vi "Move To Position According to List.vi"() -> ()   [LabVIEW 2020]
uses:
  Labview Library/Libraries/Basic Experiment/AutoTrace Element Result.ctl
  <vilib>/Analysis/coordinate.llb/3D Coordinate Conversion (Scalar).vi
  <vilib>/Utility/file.llb/Read Delimited Spreadsheet (string).vi
  Labview Library/Libraries/Read TDMS Data/Library/Read TDMS Data.lvlib
  Labview Library/Libraries/Basic Experiment/Basic Experiment.lvlib
  Labview Library/Libraries/Shift_Correction/Libraries/Shift_Correction/Shift_Correction.lvlib
  <vilib>/Analysis/NI_AALPro.lvlib
panel:
  out "Amp Difference":dbl=0.263119271037894
  out "Angle Difference (deg)":dbl=-0.09953145598427682
  out "AutoTrace Result":T1={"Pure Count"=497997.60921836324, "BackGround"=54839.90103535615, "AutoTrace File Path"=path "G:/Raw Data/AutoFocus/XY Graph/2024-03/AF XY 2024-03-21_205701.png", "Light Spot Pos"=[5.049998165058289, 143.35743224656605, 69.90496826]}
  in  "ColorCenter List Path":path=path "G:/Exp_Log/2024_02_12_ChargeDetection2/Accurate_LightSpot.csv"
  out "Table":string[][](array[string])
  in  "Index":u32=3
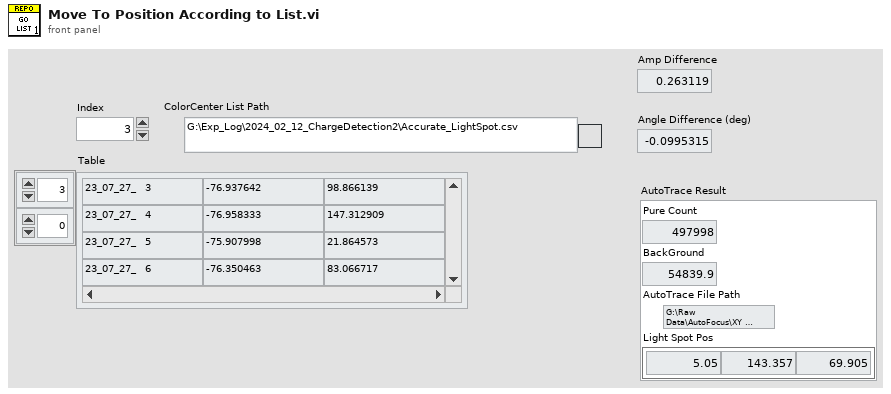
[diagram p1: front panel]
types:
  T1 = typedef "Basic Experiment.lvlib/AutoTrace Element Result.ctl" = cluster{"Pure Count":dbl, "BackGround":dbl, "AutoTrace File Path":path, "Light Spot Pos":dbl[]}
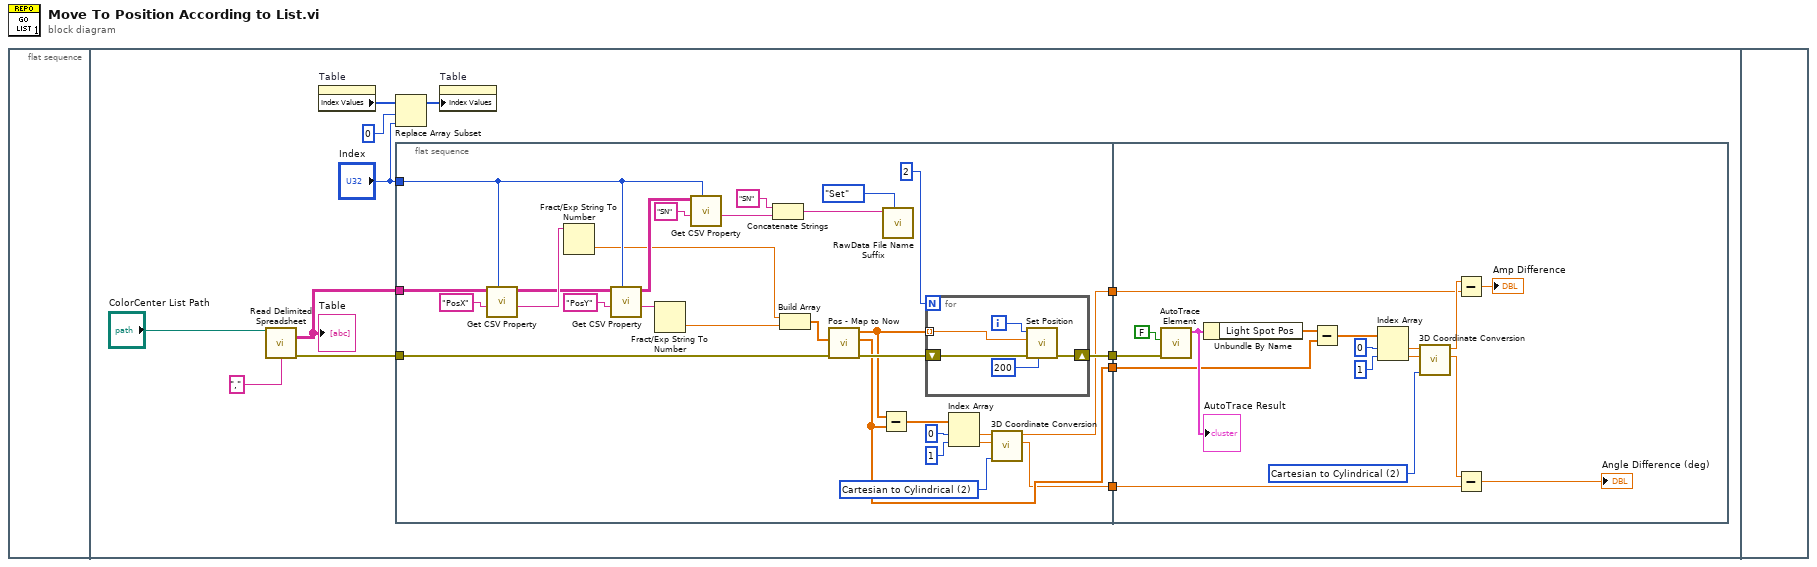
[diagram p0: block diagram]
diagram:
  n1 = flat-sequence {
    frame #0 {
    }
    frame #1 {
      n2 = call-poly <vilib>:"Read Delimited Spreadsheet.vi"("file path (dialog if empty)"="ColorCenter List Path", "delimiter (\\t)"="," ("delimiter (\\t)")) -> ("all rows"=w9:string[][], "error out"=w11:errorcluster)  [unwired: 8 in, 4 out]
      "Table" <- w9
      n3 = property on="Table" class="Arr (strict)"() -> ("Index Values"=w8:u32[])  [unwired: 2 in, 2 out]
      n4 = Replace Array Subset(array=w8, new element="Index", index=0) -> (w6:u32[])
      n5 = flat-sequence {
        tunnel: [w23] -> w4
        tunnel: w11 -> [w25]
        tunnel: "Index" -> [w34]
        tunnel: w9 -> [w41]
        tunnel: [w15] -> w3
        tunnel: [w14] -> w2
        tunnel: [w13] -> w1
        tunnel: w4 -> [w64]
        tunnel: w3 -> [w60]
        tunnel: w2 -> [w52]
        tunnel: w1 -> [w50]
        frame #0 {
          w16 = u16 2 items=["Cartesian to Spherical", "Spherical to Cartesian", "Cartesian to Cylindrical", "Cylindrical to Cartesian", "Spherical to Cylindrical", "Cylindrical to Spherical"] ("conversion type")
          n6 = call "Get CSV Property.vi"("Index"=w34, "Property Name"="PosX", "csv"=w41) -> ("Property value"=w40:string, "csv output"=w39:string[][])  [unwired: 7 in]
          n7 = Fract/Exp String To Number(string=w40) -> (number=w29:dbl)  [unwired: 3 in, 1 out]
          n8 = call "Get CSV Property.vi"("Index"=w34, "Property Name"="PosY", "csv"=w39) -> ("Property value"=w38:string, "csv output"=w36:string[][])  [unwired: 7 in]
          n9 = Fract/Exp String To Number(string=w38) -> (number=w28:dbl)  [unwired: 3 in, 1 out]
          n10 = call "Get CSV Property.vi"("Index"=w34, "Property Name"="SN", "csv"=w36) -> ("Property value"=w31:string)  [unwired: 7 in, 1 out]
          n11 = Concatenate Strings("SN" ("string"), w31) -> (w30:string)
          n12 = Build Array(w29, w28) -> (w26:dbl[])
          n13 = call "Pos - Map to Now.vi"("error in"=w25, "Goal Map Position"=w26) -> ("error out"=w24:errorcluster, "Marker Position Now"=w15:dbl[], "Goal Now Position"=w20:dbl[])  [unwired: 6 in, 1 out]
          n14 = Subtract(x=w20, y=w15) -> (x-y=w19:dbl[])
          n15 = call "RawData File Name Suffix.vi"("Mode"=enum16{"Set", "Get"}."Set", "Suffix"=w30) -> ()  [unwired: 9 in, 1 out]
          n16 = for {
            N: 2 -> [_]
            tunnel: w20 -> [w47] mode=indexing
            shift-right: [w45] -> w23
            shift-left: w24 -> [w44]
            i -> [w46]
            n17 = call "Set Position.vi"("Idle After Moving (ms)"=200, "error in"=w44, "Position"=w47, "Axis"=w46) -> ("error out"=w45:errorcluster)  [unwired: 7 in]
          }
          n18 = Index Array(array=w19, index #1=0 ("index"), index #2=1 ("index")) -> (element #1=w18:dbl, element #2=w17:dbl)
          n19 = call-poly <vilib>:"3D Coordinate Conversion.vi"("conversion type"=w16, "axis 2"=w17, "axis 1"=w18) -> ("axis 2 out"=w13:dbl, "axis 1 out"=w14:dbl)  [unwired: 5 in, 2 out]
        }
        frame #1 {
          w59 = u16 2 items=["Cartesian to Spherical", "Spherical to Cartesian", "Cartesian to Cylindrical", "Cylindrical to Cartesian", "Spherical to Cylindrical", "Cylindrical to Spherical"] ("conversion type")
          n20 = call "AutoTrace Element.vi"("error in (no error)"=w64, "Need Correct Count?(T)"=FALSE) -> ("AutoTrace Result"=w62:T1)  [unwired: 8 in, 1 out]
          "AutoTrace Result" <- w62
          n21 = Unbundle By Name(w62) -> ("Light Spot Pos"=w61:dbl[])
          n22 = Subtract(x=w61, y=w60) -> (x-y=w54:dbl[])
          n23 = Index Array(array=w54, index #1=0 ("index"), index #2=1 ("index")) -> (element #1=w57:dbl, element #2=w58:dbl)
          n24 = call-poly <vilib>:"3D Coordinate Conversion.vi"("conversion type"=w59, "axis 2"=w58, "axis 1"=w57) -> ("axis 2 out"=w51:dbl, "axis 1 out"=w53:dbl)  [unwired: 5 in, 2 out]
          n25 = Subtract(x=w53, y=w52) -> (x-y=→"Amp Difference":dbl)
          n26 = Subtract(x=w51, y=w50) -> (x-y=→"Angle Difference (deg)":dbl)
        }
      }
      n27 = property on="Table" class="Arr (strict)"("Index Values"=w6) -> ()  [unwired: 2 in, 2 out]
    }
    frame #2 {
    }
  }
